vi "LinearInterpolate.vi"(10 "Config":T1, 11 "Value":dbl) -> (3 "Output":dbl)   [LabVIEW 2016]
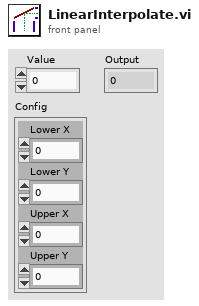
[diagram p1: front panel]
types:
  T1 = cluster{"Lower X":dbl, "Lower Y":dbl, "Upper X":dbl, "Upper Y":dbl}
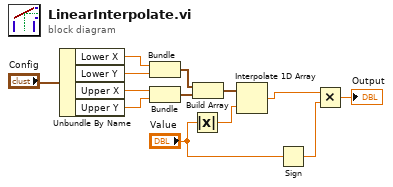
[diagram p0: block diagram]
diagram:
  n1 = Unbundle By Name("Config") -> ("Lower X"=w12:dbl, "Lower Y"=w11:dbl, "Upper X"=w10:dbl, "Upper Y"=w9:dbl)
  n2 = Bundle("Lower X"=w12, "Lower Y"=w11) -> (w8:cluster{"Lower X":dbl, "Lower Y":dbl})  [unwired: 1 in]
  n3 = Bundle("Upper X"=w10, "Upper Y"=w9) -> (w7:cluster{"Upper X":dbl, "Upper Y":dbl})  [unwired: 1 in]
  n4 = Absolute Value(x="Value") -> (abs(x)=w3:dbl)
  n5 = Build Array(w8, w7) -> (w6:cluster{"Upper X":dbl, "Upper Y":dbl}[])
  n6 = Interpolate 1D Array(1:w3, 2:w6) -> (0:w1:dbl)
  n7 = Sign(1:"Value") -> (0:w5:dbl)
  n8 = Multiply(x=w1, y=w5) -> (x*y=→"Output":dbl)
